vi "SO55 Ion Source Main.vi"() -> ()   [LabVIEW 2013]
panel:
  out "AnodeCurrentInd":dbl format="%#.3g"
  out "Anode Current":dbl(knob) scale=0.0..10.0
  out "GasInd":dbl format="%#.3g"
  out "Gasmeter":dbl(knob) scale=0.0..40.0
  in  "Gas":dbl(knob) min=0.0 max=40.0 step=0.1 scale=0.0..40.0
  in  "ExitBtn":bool
  in  "SetBtn":bool
  out "AnodeInd":dbl format="%#.3g"
  out "Anodemeter":dbl(knob) scale=0.0..250.0 scale format="%-#3.3p"
  in  "Anode":dbl(knob) min=0.0 max=250.0 step=1.0 scale=0.0..250.0
  out "OvenInd":dbl format="%#.3g"
  out "MagInd":dbl format="%#.3g"
  out "FilInd":dbl format="%#.3g"
  out "Ovenmeter":dbl(knob) scale=0.0..40.0
  out "Magmeter":dbl(knob) scale=0.0..40.0
  out "Filmeter":dbl(knob) scale=0.0..40.0 scale format="%-#3.3p"
  in  "Oven":dbl(knob) min=0.0 max=40.0 step=0.1 scale=0.0..40.0
  in  "Mag":dbl(knob) min=0.0 max=30.0 step=0.1 scale=0.0..40.0
  in  "Fil":dbl(knob) min=0.0 max=40.0 step=0.1 scale=0.0..40.0
  # "Magnet"
  # "Oven"
  # "Gas"
  # "Anode"
  # "Filament"
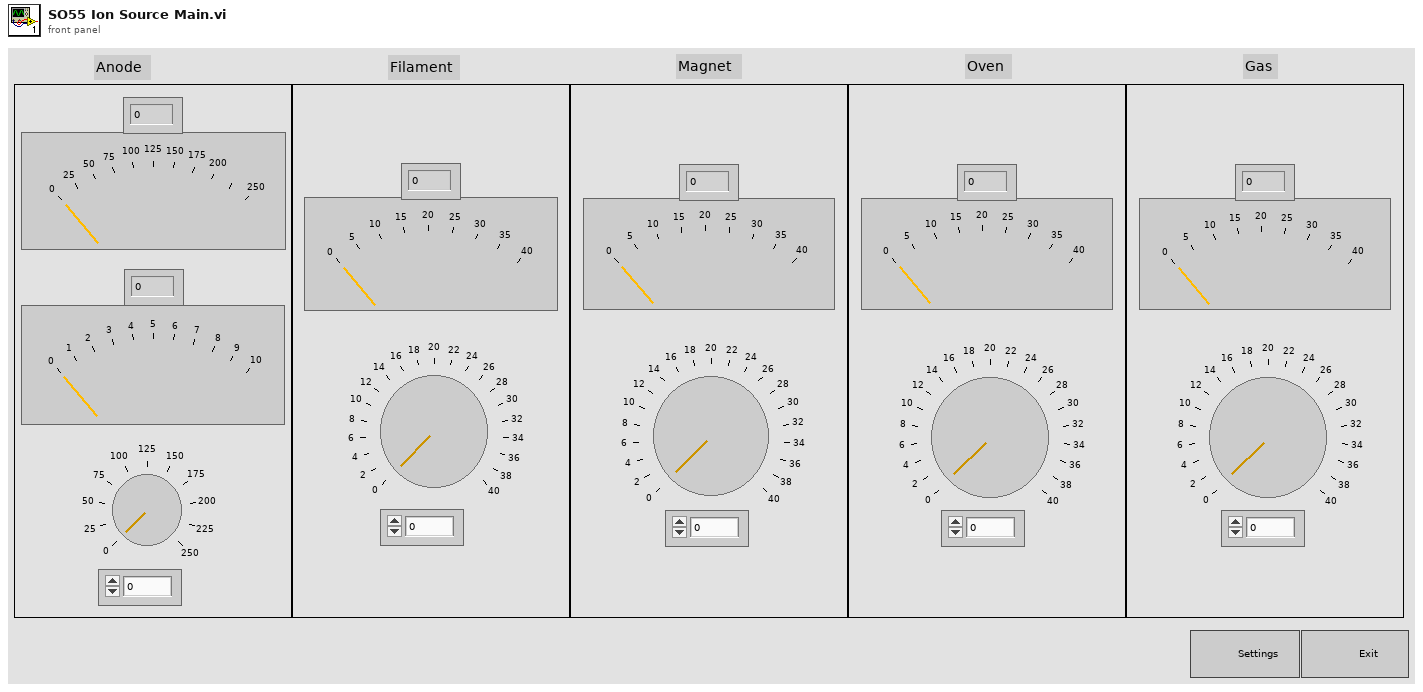
[diagram p1: front panel]
types:
  T1 = typedef "SO55 Settings Cluster.ctl" = cluster{"Input":cluster{"Anode Input Channel":tag, "Filament Input Channel":tag, "Magnet Input Channel":tag, "Oven Input Channel":tag, "Gas Input Channel":tag, "Input Rate":dbl, "Anode Current Input Channel":tag}, "Output":cluster{"Anode":cluster{"Anode Output Channel":tag, "Anode Step":dbl}, "Filament":cluster{"Filament Output Channel":tag, "Filament Step":dbl}, "Magnet":cluster{"Magnet Output Channel":tag, "Magnet Step":dbl}, "Oven":cluster{"Oven Output Channel":tag, "Oven Step":dbl}, "Gas":cluster{"Gas Output Channel":tag, "Gas Step":dbl}, "Output Rate":dbl}}
  T2 = enum8{"Enabled", "Disabled", "Disabled and Grayed Out"}
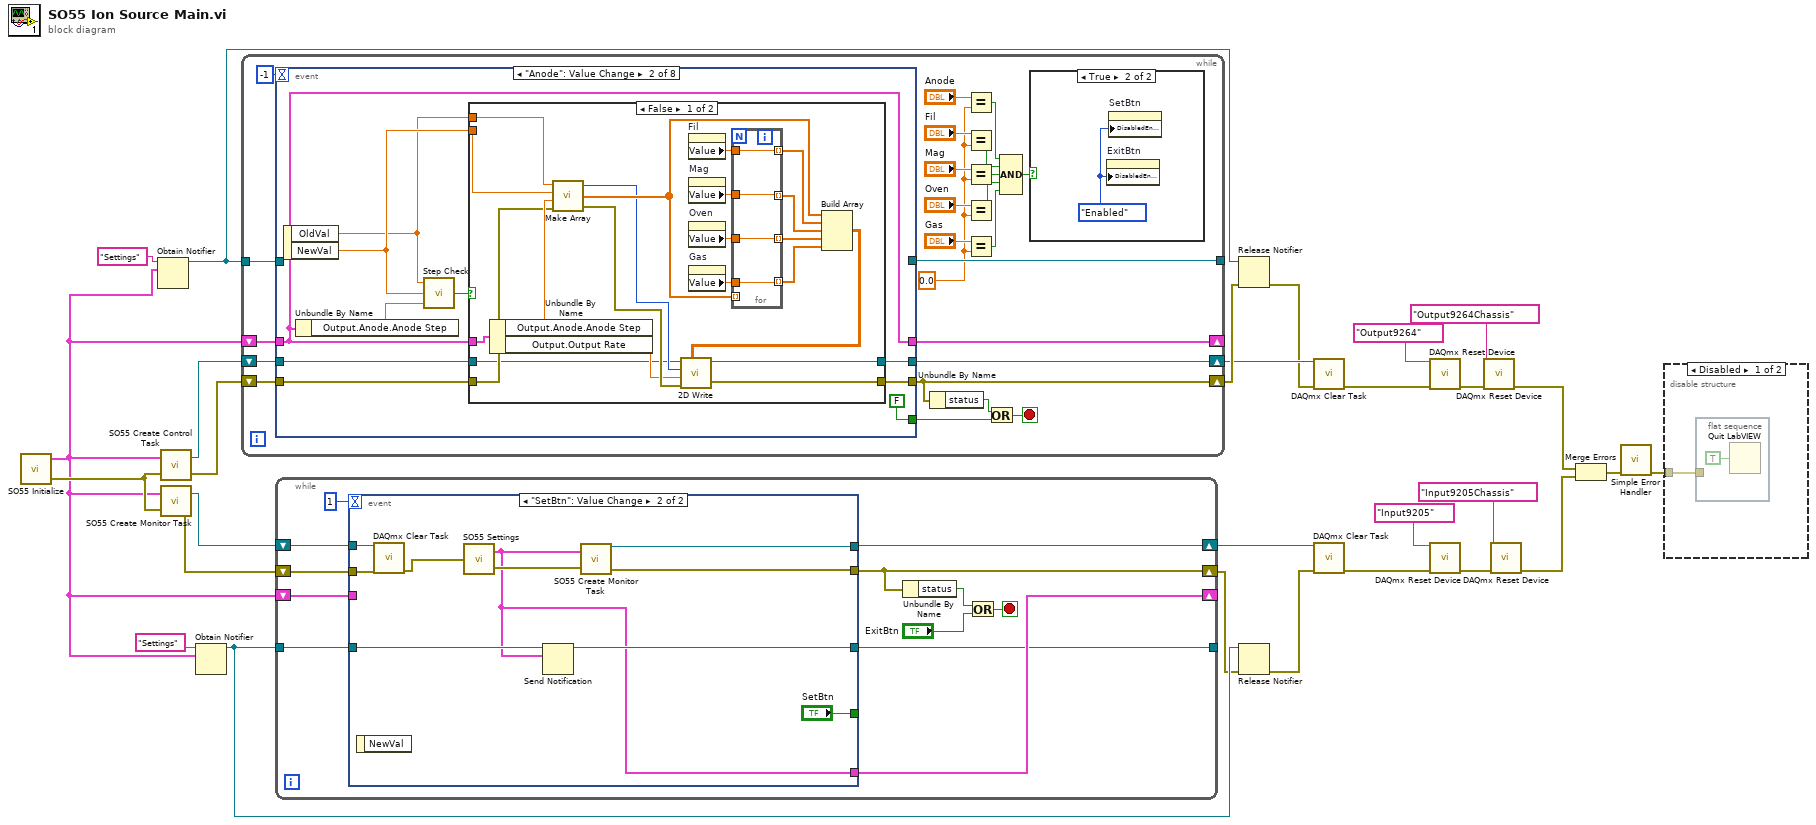
[diagram p0: block diagram]
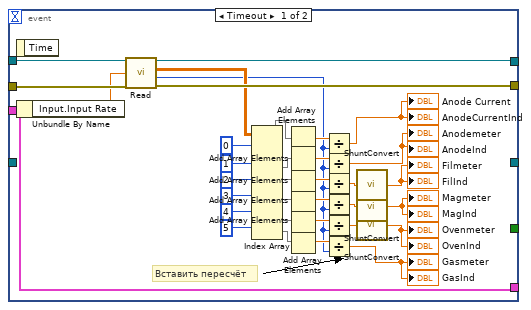
[diagram p3: hidden frame]
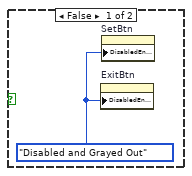
[diagram p4: hidden frame]
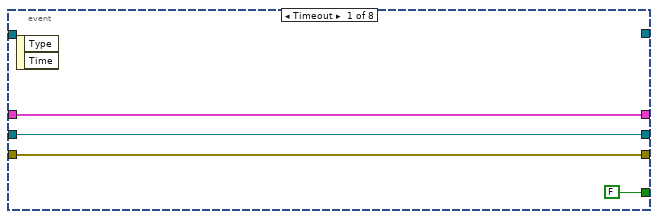
[diagram p5: hidden frame]
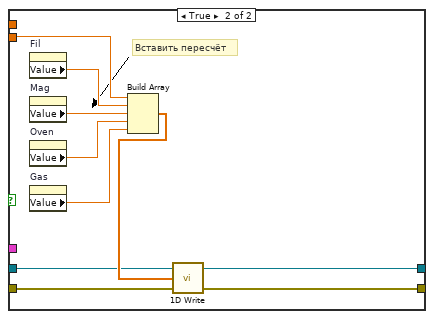
[diagram p6: hidden frame]
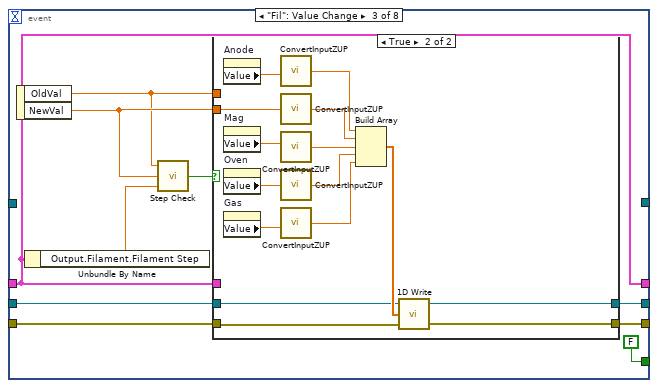
[diagram p7: hidden frame]
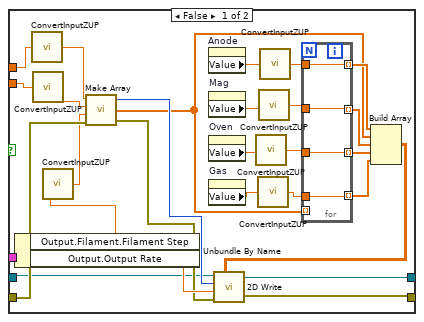
[diagram p8: hidden frame]
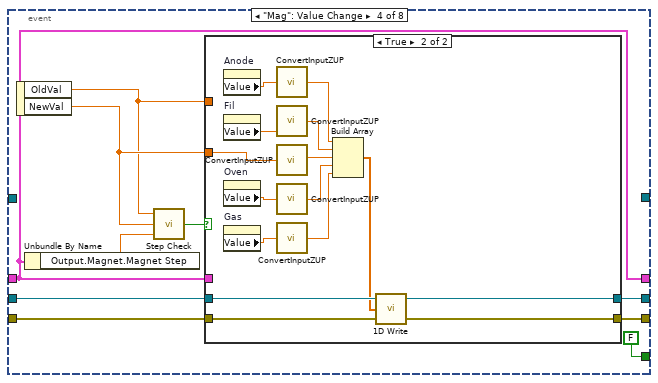
[diagram p9: hidden frame]
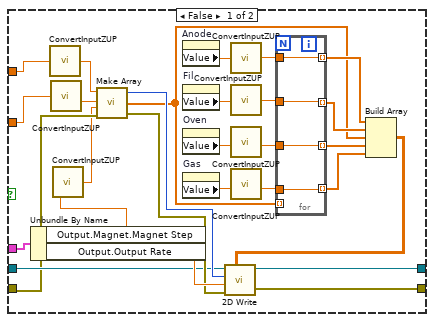
[diagram p10: hidden frame]
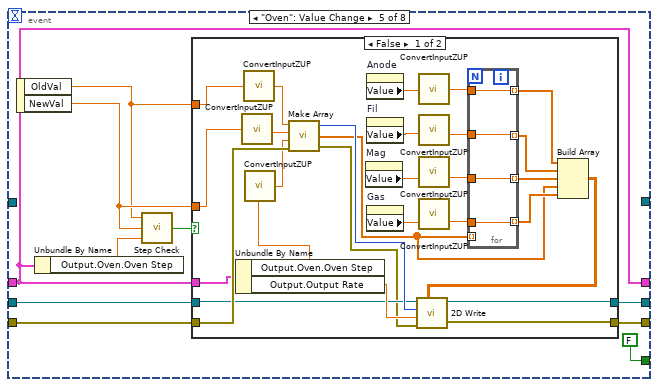
[diagram p11: hidden frame]
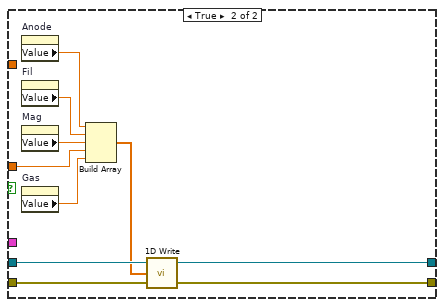
[diagram p12: hidden frame]
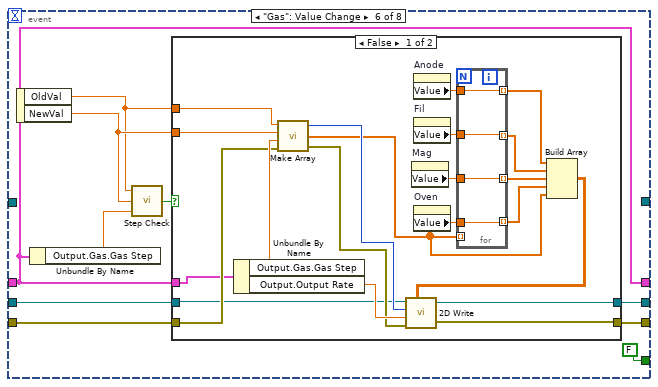
[diagram p13: hidden frame]
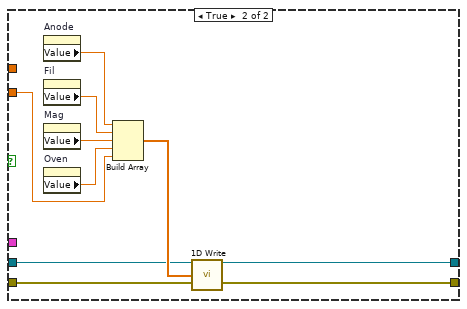
[diagram p14: hidden frame]
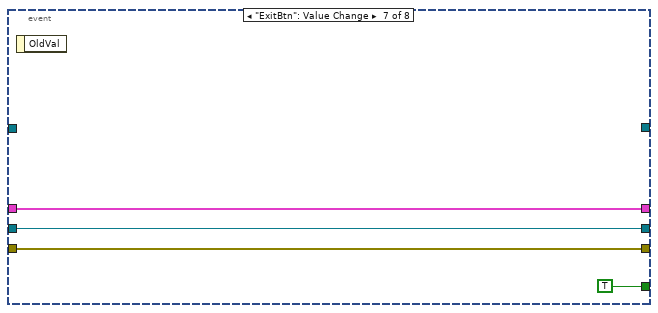
[diagram p15: hidden frame]
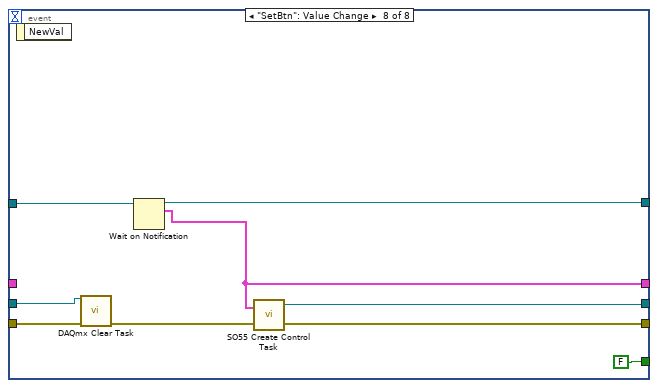
[diagram p16: hidden frame]
diagram:
  n1 = call "SO55 Initialize.vi"() -> ("error out"=w28:errorcluster, "Settings Out"=w1:T1)  [unwired: 1 in]
  n2 = Obtain Notifier(name (unnamed)="Settings", notification data type=w1) -> (notifier out=w3:refnum<notifier>)  [unwired: 2 in, 2 out]
  n3 = call "SO55 Create Control Task.vi"("error in"=w28, "Output"=w1) -> ("error out"=w24:errorcluster, "task out"=w25:refnum<k21>)
  n4 = call "SO55 Create Monitor Task.vi"("error in"=w28, "Input"=w1) -> ("error out"=w26:errorcluster, "task out"=w27:refnum<k21>)
  n5 = Obtain Notifier(name (unnamed)="Settings", notification data type=w1) -> (notifier out=w4:refnum<notifier>)  [unwired: 2 in, 2 out]
  n6 = while {
    shift-right: [w46] -> w21
    shift-left: w24 -> [w49]
    shift-right: [w51] -> w20
    shift-left: w25 -> [w50]
    shift-right: [w47] -> _
    shift-left: w1 -> [w48]
    tunnel: w3 -> [w42]
    tunnel: [w41] -> _
    stop <- w43 stop-if-true
    w35 = 0.0
    n7 = event shown="[1] \"Anode\": Value Change" {
      selector: _ -> [_ _ _ _ _ _ _ _]
      dyn-events: _ -> [_ _ _ _ _ _ _ _]
      timeout: -1 -> [_ _ _ _ _ _ _ _]
      tunnel: [w58 w66 w111 w165 w222 w274 w316 w321] -> w51
      tunnel: w50 -> [w58 w68 w113 w167 w224 w276 w316 w325]
      tunnel: [w57 w65 w110 w164 w221 w273 w315 w320] -> w46
      tunnel: w49 -> [w57 w67 w112 w166 w223 w275 w315 w326]
      tunnel: [w56 w59 w104 w161 w218 w270 w317 w319] -> w47
      tunnel: w48 -> [w56 w59 w104 w161 w218 w270 w317 _]
      tunnel: [FALSE FALSE FALSE FALSE FALSE FALSE TRUE FALSE] -> w44
      tunnel: w42 -> [_ _ _ _ _ _ _ w324]
      tunnel: [_ _ _ _ _ _ _ w323] -> w41
      event Timeout {
        n8 = event-data() -> ()  [unwired: 1 in, 2 out]
      }
      event "Anode": Value Change {
        n9 = event-data() -> ("OldVal"=w60:dbl, "NewVal"=w63:dbl)  [unwired: 1 in]
        n10 = Unbundle By Name(w59) -> ("Output.Anode.Anode Step"=w62:dbl)
        n11 = call "Step Check.vi"("Step"=w62, "New Value"=w63, "Old Value"=w60) -> ("Instant output"=w64:bool)
        n12 = case shown="False" w64 {
          tunnel: w63 -> [w87 w103]
          tunnel: w68 -> [w69 w97]
          tunnel: w67 -> [w85 w96]
          tunnel: [w71 w95] -> w66
          tunnel: [w70 w94] -> w65
          tunnel: w60 -> [w88 _]
          tunnel: w59 -> [w89 _]
          frame False {
            n13 = Unbundle By Name(w89) -> ("Output.Anode.Anode Step"=w86:dbl, "Output.Output Rate"=w72:dbl)
            n14 = call "Make Array.vi"("Error In"=w85, "Step"=w86, "New"=w87, "Old"=w88) -> ("Error Out"=w74:errorcluster, "Array"=w76:dbl[], "Samples"=w73:i32)
            n15 = property on="Fil" class="Knob (strict)"() -> ("Value"=w84:dbl)  [unwired: 2 in, 2 out]
            n16 = property on="Mag" class="Knob (strict)"() -> ("Value"=w83:dbl)  [unwired: 2 in, 2 out]
            n17 = property on="Oven" class="Knob (strict)"() -> ("Value"=w82:dbl)  [unwired: 2 in, 2 out]
            n18 = property on="Gas" class="Knob (strict)"() -> ("Value"=w81:dbl)  [unwired: 2 in, 2 out]
            n19 = for {
              tunnel: w84 -> [w93]
              tunnel: w83 -> [w92]
              tunnel: w76 -> [_] mode=indexing
              tunnel: w82 -> [w91]
              tunnel: w81 -> [w90]
              tunnel: [w93] -> w77 mode=indexing
              tunnel: [w92] -> w78 mode=indexing
              tunnel: [w91] -> w79 mode=indexing
              tunnel: [w90] -> w80 mode=indexing
            }
            n20 = Build Array(w76, w77, w78, w79, w80) -> (w75:dbl[][])
            n21 = call "2D Write.vi"("Task"=w69, "samples per channel"=w73, "rate"=w72, "Error In"=w74, "data"=w75) -> ("task out"=w71:refnum<k21>, "Error Out"=w70:errorcluster)
          }
          frame True {
            # "Вставить пересчёт"
            n22 = property on="Fil" class="Knob (strict)"() -> ("Value"=w99:dbl)  [unwired: 2 in, 2 out]
            n23 = property on="Mag" class="Knob (strict)"() -> ("Value"=w102:dbl)  [unwired: 2 in, 2 out]
            n24 = property on="Oven" class="Knob (strict)"() -> ("Value"=w101:dbl)  [unwired: 2 in, 2 out]
            n25 = property on="Gas" class="Knob (strict)"() -> ("Value"=w100:dbl)  [unwired: 2 in, 2 out]
            n26 = Build Array(w103, w99, w102, w101, w100) -> (w98:dbl[])
            n27 = call "1D Write.vi"("error in (no error)"=w96, "Data Array"=w98, "Task in"=w97) -> ("error out"=w94:errorcluster, "Task out"=w95:refnum<k21>)
          }
        }
      }
      event "Fil": Value Change {
        n28 = event-data() -> ("OldVal"=w105:dbl, "NewVal"=w107:dbl)  [unwired: 1 in]
        n29 = Unbundle By Name(w104) -> ("Output.Filament.Filament Step"=w108:dbl)
        n30 = call "Step Check.vi"("Step"=w108, "New Value"=w107, "Old Value"=w105) -> ("Instant output"=w109:bool)
        n31 = case shown="True" w109 {
          tunnel: w107 -> [w125 w153]
          tunnel: w113 -> [w130 w159]
          tunnel: w112 -> [w133 w158]
          tunnel: [w129 w157] -> w111
          tunnel: [w131 w156] -> w110
          tunnel: w104 -> [w128 _]
          tunnel: w105 -> [w127 _]
          frame False {
            n32 = Unbundle By Name(w128) -> ("Output.Filament.Filament Step"=w123:dbl, "Output.Output Rate"=w136:dbl)
            n33 = call "ConvertInputZUP.vi"("Current"=w127) -> ("ZUP input voltage"=w126:dbl)
            n34 = call "ConvertInputZUP.vi"("Current"=w125) -> ("ZUP input voltage"=w124:dbl)
            n35 = call "ConvertInputZUP.vi"("Current"=w123) -> ("ZUP input voltage"=w122:dbl)
            n36 = call "Make Array.vi"("Error In"=w133, "Step"=w122, "New"=w124, "Old"=w126) -> ("Error Out"=w132:errorcluster, "Array"=w134:dbl[], "Samples"=w137:i32)
            n37 = property on="Anode" class="Knob (strict)"() -> ("Value"=w114:dbl)  [unwired: 2 in, 2 out]
            n38 = property on="Mag" class="Knob (strict)"() -> ("Value"=w117:dbl)  [unwired: 2 in, 2 out]
            n39 = property on="Oven" class="Knob (strict)"() -> ("Value"=w119:dbl)  [unwired: 2 in, 2 out]
            n40 = property on="Gas" class="Knob (strict)"() -> ("Value"=w121:dbl)  [unwired: 2 in, 2 out]
            n41 = call "ConvertInputZUP.vi"("Current"=w119) -> ("ZUP input voltage"=w118:dbl)
            n42 = call "ConvertInputZUP.vi"("Current"=w121) -> ("ZUP input voltage"=w120:dbl)
            n43 = call "ConvertInputZUP.vi"("Current"=w117) -> ("ZUP input voltage"=w116:dbl)
            n44 = call "ConvertInputZUP.vi"("Current"=w114) -> ("ZUP input voltage"=w115:dbl)
            n45 = for {
              tunnel: w115 -> [w145]
              tunnel: w116 -> [w144]
              tunnel: w134 -> [_] mode=indexing
              tunnel: w118 -> [w143]
              tunnel: w120 -> [w142]
              tunnel: [w145] -> w135 mode=indexing
              tunnel: [w144] -> w139 mode=indexing
              tunnel: [w143] -> w140 mode=indexing
              tunnel: [w142] -> w141 mode=indexing
            }
            n46 = Build Array(w135, w134, w139, w140, w141) -> (w138:dbl[][])
            n47 = call "2D Write.vi"("Task"=w130, "samples per channel"=w137, "rate"=w136, "Error In"=w132, "data"=w138) -> ("task out"=w129:refnum<k21>, "Error Out"=w131:errorcluster)
          }
          frame True {
            n48 = property on="Anode" class="Knob (strict)"() -> ("Value"=w155:dbl)  [unwired: 2 in, 2 out]
            n49 = property on="Mag" class="Knob (strict)"() -> ("Value"=w151:dbl)  [unwired: 2 in, 2 out]
            n50 = property on="Oven" class="Knob (strict)"() -> ("Value"=w149:dbl)  [unwired: 2 in, 2 out]
            n51 = property on="Gas" class="Knob (strict)"() -> ("Value"=w147:dbl)  [unwired: 2 in, 2 out]
            n52 = call "ConvertInputZUP.vi"("Current"=w155) -> ("ZUP input voltage"=w154:dbl)
            n53 = call "ConvertInputZUP.vi"("Current"=w153) -> ("ZUP input voltage"=w152:dbl)
            n54 = call "ConvertInputZUP.vi"("Current"=w151) -> ("ZUP input voltage"=w150:dbl)
            n55 = call "ConvertInputZUP.vi"("Current"=w149) -> ("ZUP input voltage"=w148:dbl)
            n56 = call "ConvertInputZUP.vi"("Current"=w147) -> ("ZUP input voltage"=w146:dbl)
            n57 = Build Array(w154, w152, w150, w148, w146) -> (w160:dbl[])
            n58 = call "1D Write.vi"("error in (no error)"=w158, "Data Array"=w160, "Task in"=w159) -> ("error out"=w156:errorcluster, "Task out"=w157:refnum<k21>)
          }
        }
      }
      event "Mag": Value Change {
        n59 = event-data() -> ("OldVal"=w162:dbl, "NewVal"=w168:dbl)  [unwired: 1 in]
        n60 = Unbundle By Name(w161) -> ("Output.Magnet.Magnet Step"=w169:dbl)
        n61 = call "Step Check.vi"("Step"=w169, "New Value"=w168, "Old Value"=w162) -> ("Instant output"=w170:bool)
        n62 = case shown="True" w170 {
          tunnel: w168 -> [w181 w207]
          tunnel: w167 -> [w189 w217]
          tunnel: w166 -> [w188 w216]
          tunnel: [w191 w215] -> w165
          tunnel: [w190 w214] -> w164
          tunnel: w162 -> [w184 _]
          tunnel: w161 -> [w185 _]
          frame False {
            n63 = Unbundle By Name(w185) -> ("Output.Magnet.Magnet Step"=w180:dbl, "Output.Output Rate"=w194:dbl)
            n64 = call "ConvertInputZUP.vi"("Current"=w184) -> ("ZUP input voltage"=w183:dbl)
            n65 = call "ConvertInputZUP.vi"("Current"=w181) -> ("ZUP input voltage"=w182:dbl)
            n66 = call "ConvertInputZUP.vi"("Current"=w180) -> ("ZUP input voltage"=w179:dbl)
            n67 = call "Make Array.vi"("Error In"=w188, "Step"=w179, "New"=w182, "Old"=w183) -> ("Error Out"=w192:errorcluster, "Array"=w186:dbl[], "Samples"=w195:i32)
            n68 = property on="Anode" class="Knob (strict)"() -> ("Value"=w177:dbl)  [unwired: 2 in, 2 out]
            n69 = property on="Fil" class="Knob (strict)"() -> ("Value"=w176:dbl)  [unwired: 2 in, 2 out]
            n70 = property on="Oven" class="Knob (strict)"() -> ("Value"=w174:dbl)  [unwired: 2 in, 2 out]
            n71 = property on="Gas" class="Knob (strict)"() -> ("Value"=w172:dbl)  [unwired: 2 in, 2 out]
            n72 = call "ConvertInputZUP.vi"("Current"=w177) -> ("ZUP input voltage"=w178:dbl)
            n73 = call "ConvertInputZUP.vi"("Current"=w176) -> ("ZUP input voltage"=w175:dbl)
            n74 = call "ConvertInputZUP.vi"("Current"=w174) -> ("ZUP input voltage"=w173:dbl)
            n75 = call "ConvertInputZUP.vi"("Current"=w172) -> ("ZUP input voltage"=w171:dbl)
            n76 = for {
              tunnel: w178 -> [w202]
              tunnel: w175 -> [w201]
              tunnel: w186 -> [_] mode=indexing
              tunnel: w173 -> [w200]
              tunnel: w171 -> [w199]
              tunnel: [w202] -> w193 mode=indexing
              tunnel: [w201] -> w187 mode=indexing
              tunnel: [w200] -> w197 mode=indexing
              tunnel: [w199] -> w198 mode=indexing
            }
            n77 = Build Array(w193, w187, w186, w197, w198) -> (w196:dbl[][])
            n78 = call "2D Write.vi"("Task"=w189, "samples per channel"=w195, "rate"=w194, "Error In"=w192, "data"=w196) -> ("task out"=w191:refnum<k21>, "Error Out"=w190:errorcluster)
          }
          frame True {
            n79 = property on="Anode" class="Knob (strict)"() -> ("Value"=w212:dbl)  [unwired: 2 in, 2 out]
            n80 = property on="Fil" class="Knob (strict)"() -> ("Value"=w210:dbl)  [unwired: 2 in, 2 out]
            n81 = property on="Oven" class="Knob (strict)"() -> ("Value"=w206:dbl)  [unwired: 2 in, 2 out]
            n82 = property on="Gas" class="Knob (strict)"() -> ("Value"=w204:dbl)  [unwired: 2 in, 2 out]
            n83 = call "ConvertInputZUP.vi"("Current"=w212) -> ("ZUP input voltage"=w211:dbl)
            n84 = call "ConvertInputZUP.vi"("Current"=w210) -> ("ZUP input voltage"=w209:dbl)
            n85 = call "ConvertInputZUP.vi"("Current"=w207) -> ("ZUP input voltage"=w208:dbl)
            n86 = call "ConvertInputZUP.vi"("Current"=w206) -> ("ZUP input voltage"=w205:dbl)
            n87 = call "ConvertInputZUP.vi"("Current"=w204) -> ("ZUP input voltage"=w203:dbl)
            n88 = Build Array(w211, w209, w208, w205, w203) -> (w213:dbl[])
            n89 = call "1D Write.vi"("error in (no error)"=w216, "Data Array"=w213, "Task in"=w217) -> ("error out"=w214:errorcluster, "Task out"=w215:refnum<k21>)
          }
        }
      }
      event "Oven": Value Change {
        n90 = event-data() -> ("OldVal"=w219:dbl, "NewVal"=w225:dbl)  [unwired: 1 in]
        n91 = Unbundle By Name(w218) -> ("Output.Oven.Oven Step"=w226:dbl)
        n92 = call "Step Check.vi"("Step"=w226, "New Value"=w225, "Old Value"=w219) -> ("Instant output"=w227:bool)
        n93 = case shown="False" w227 {
          tunnel: w225 -> [w238 w268]
          tunnel: w224 -> [w246 w264]
          tunnel: w223 -> [w247 w263]
          tunnel: [w249 w262] -> w222
          tunnel: [w248 w261] -> w221
          tunnel: w219 -> [w240 _]
          tunnel: w218 -> [w245 _]
          frame False {
            n94 = Unbundle By Name(w245) -> ("Output.Oven.Oven Step"=w236:dbl, "Output.Output Rate"=w252:dbl)
            n95 = call "ConvertInputZUP.vi"("Current"=w238) -> ("ZUP input voltage"=w239:dbl)
            n96 = call "ConvertInputZUP.vi"("Current"=w240) -> ("ZUP input voltage"=w241:dbl)
            n97 = call "ConvertInputZUP.vi"("Current"=w236) -> ("ZUP input voltage"=w237:dbl)
            n98 = call "Make Array.vi"("Error In"=w247, "Step"=w237, "New"=w239, "Old"=w241) -> ("Error Out"=w244:errorcluster, "Array"=w242:dbl[], "Samples"=w253:i32)
            n99 = property on="Mag" class="Knob (strict)"() -> ("Value"=w231:dbl)  [unwired: 2 in, 2 out]
            n100 = property on="Anode" class="Knob (strict)"() -> ("Value"=w234:dbl)  [unwired: 2 in, 2 out]
            n101 = property on="Fil" class="Knob (strict)"() -> ("Value"=w233:dbl)  [unwired: 2 in, 2 out]
            n102 = property on="Gas" class="Knob (strict)"() -> ("Value"=w230:dbl)  [unwired: 2 in, 2 out]
            n103 = call "ConvertInputZUP.vi"("Current"=w234) -> ("ZUP input voltage"=w235:dbl)
            n104 = call "ConvertInputZUP.vi"("Current"=w233) -> ("ZUP input voltage"=w232:dbl)
            n105 = call "ConvertInputZUP.vi"("Current"=w231) -> ("ZUP input voltage"=w228:dbl)
            n106 = call "ConvertInputZUP.vi"("Current"=w230) -> ("ZUP input voltage"=w229:dbl)
            n107 = for {
              tunnel: w235 -> [w259]
              tunnel: w232 -> [w258]
              tunnel: w242 -> [_] mode=indexing
              tunnel: w228 -> [w257]
              tunnel: w229 -> [w256]
              tunnel: [w259] -> w251 mode=indexing
              tunnel: [w258] -> w250 mode=indexing
              tunnel: [w257] -> w243 mode=indexing
              tunnel: [w256] -> w255 mode=indexing
            }
            n108 = Build Array(w251, w250, w243, w242, w255) -> (w254:dbl[][])
            n109 = call "2D Write.vi"("Task"=w246, "samples per channel"=w253, "rate"=w252, "Error In"=w244, "data"=w254) -> ("task out"=w249:refnum<k21>, "Error Out"=w248:errorcluster)
          }
          frame True {
            n110 = property on="Anode" class="Knob (strict)"() -> ("Value"=w265:dbl)  [unwired: 2 in, 2 out]
            n111 = property on="Fil" class="Knob (strict)"() -> ("Value"=w266:dbl)  [unwired: 2 in, 2 out]
            n112 = property on="Mag" class="Knob (strict)"() -> ("Value"=w267:dbl)  [unwired: 2 in, 2 out]
            n113 = property on="Gas" class="Knob (strict)"() -> ("Value"=w269:dbl)  [unwired: 2 in, 2 out]
            n114 = Build Array(w265, w266, w267, w268, w269) -> (w260:dbl[])
            n115 = call "1D Write.vi"("error in (no error)"=w263, "Data Array"=w260, "Task in"=w264) -> ("error out"=w261:errorcluster, "Task out"=w262:refnum<k21>)
          }
        }
      }
      event "Gas": Value Change {
        n116 = event-data() -> ("OldVal"=w271:dbl, "NewVal"=w277:dbl)  [unwired: 1 in]
        n117 = Unbundle By Name(w270) -> ("Output.Gas.Gas Step"=w278:dbl)
        n118 = call "Step Check.vi"("Step"=w278, "New Value"=w277, "Old Value"=w271) -> ("Instant output"=w279:bool)
        n119 = case shown="False" w279 {
          tunnel: w277 -> [w285 w310]
          tunnel: w276 -> [w288 w308]
          tunnel: w275 -> [w289 w307]
          tunnel: [w291 w306] -> w274
          tunnel: [w290 w305] -> w273
          tunnel: w270 -> [w287 _]
          tunnel: w271 -> [w286 _]
          frame False {
            n120 = Unbundle By Name(w287) -> ("Output.Gas.Gas Step"=w300:dbl, "Output.Output Rate"=w297:dbl)
            n121 = call "Make Array.vi"("Error In"=w289, "Step"=w300, "New"=w285, "Old"=w286) -> ("Error Out"=w294:errorcluster, "Array"=w280:dbl[], "Samples"=w298:i32)
            n122 = property on="Mag" class="Knob (strict)"() -> ("Value"=w283:dbl)  [unwired: 2 in, 2 out]
            n123 = property on="Anode" class="Knob (strict)"() -> ("Value"=w296:dbl)  [unwired: 2 in, 2 out]
            n124 = property on="Fil" class="Knob (strict)"() -> ("Value"=w293:dbl)  [unwired: 2 in, 2 out]
            n125 = property on="Oven" class="Knob (strict)"() -> ("Value"=w284:dbl)  [unwired: 2 in, 2 out]
            n126 = for {
              tunnel: w296 -> [w304]
              tunnel: w293 -> [w303]
              tunnel: w280 -> [_] mode=indexing
              tunnel: w283 -> [w302]
              tunnel: w284 -> [w301]
              tunnel: [w304] -> w295 mode=indexing
              tunnel: [w303] -> w292 mode=indexing
              tunnel: [w302] -> w282 mode=indexing
              tunnel: [w301] -> w281 mode=indexing
            }
            n127 = Build Array(w295, w292, w282, w281, w280) -> (w299:dbl[][])
            n128 = call "2D Write.vi"("Task"=w288, "samples per channel"=w298, "rate"=w297, "Error In"=w294, "data"=w299) -> ("task out"=w291:refnum<k21>, "Error Out"=w290:errorcluster)
          }
          frame True {
            n129 = property on="Anode" class="Knob (strict)"() -> ("Value"=w313:dbl)  [unwired: 2 in, 2 out]
            n130 = property on="Fil" class="Knob (strict)"() -> ("Value"=w314:dbl)  [unwired: 2 in, 2 out]
            n131 = property on="Mag" class="Knob (strict)"() -> ("Value"=w312:dbl)  [unwired: 2 in, 2 out]
            n132 = property on="Oven" class="Knob (strict)"() -> ("Value"=w311:dbl)  [unwired: 2 in, 2 out]
            n133 = Build Array(w313, w314, w312, w311, w310) -> (w309:dbl[])
            n134 = call "1D Write.vi"("error in (no error)"=w307, "Data Array"=w309, "Task in"=w308) -> ("error out"=w305:errorcluster, "Task out"=w306:refnum<k21>)
          }
        }
      }
      event "ExitBtn": Value Change {
        n135 = event-data() -> ()  [unwired: 1 in, 1 out]
      }
      event "SetBtn": Value Change {
        n136 = event-data() -> ()  [unwired: 1 in, 1 out]
        n137 = call <vilib>:"DAQmx Clear Task.vi"("task in"=w325, "error in"=w326) -> ("error out"=w322:errorcluster)  [unwired: 13 in]
        n138 = Wait on Notification(notifier=w324) -> (notifier out=w323:refnum<notifier>, notification=w319:T1)  [unwired: 3 in, 2 out]
        n139 = call "SO55 Create Control Task.vi"("error in"=w322, "Output"=w319) -> ("error out"=w320:errorcluster, "task out"=w321:refnum<k21>)
      }
    }
    n140 = Unbundle By Name(w46) -> ("status"=w45:bool)
    n141 = Equal?(x="Anode", y=w35) -> (x = y?=w34:bool)
    n142 = Equal?(x="Fil", y=w35) -> (x = y?=w33:bool)
    n143 = Equal?(x="Mag", y=w35) -> (x = y?=w32:bool)
    n144 = Equal?(x="Oven", y=w35) -> (x = y?=w31:bool)
    n145 = Equal?(x="Gas", y=w35) -> (x = y?=w30:bool)
    n146 = Or(x=w45, y=w44) -> (x .or. y?=w43:bool)
    n147 = Compound Arithmetic op=AND(w34, w33, w32, w31, w30) -> (w29:bool)
    n148 = case shown="True" w29 {
      frame False {
        w53 = T2."Disabled and Grayed Out" ("Disabled")
        n149 = property on="ExitBtn" class="Bool"("DisabledEnum"=w53) -> ()  [unwired: 2 in, 2 out]
        n150 = property on="SetBtn" class="Bool"("DisabledEnum"=w53) -> ()  [unwired: 2 in, 2 out]
      }
      frame True {
        w54 = T2."Enabled" ("Disabled")
        n151 = property on="ExitBtn" class="Bool"("DisabledEnum"=w54) -> ()  [unwired: 2 in, 2 out]
        n152 = property on="SetBtn" class="Bool"("DisabledEnum"=w54) -> ()  [unwired: 2 in, 2 out]
      }
    }
  }
  n153 = while {
    shift-right: [w333] -> w2
    shift-left: w26 -> [w337]
    shift-right: [w335] -> w18
    shift-left: w27 -> [w338]
    shift-right: [w334] -> _
    shift-left: w1 -> [w336]
    tunnel: w4 -> [w329]
    tunnel: [w328] -> _
    stop <- w330 stop-if-true
    n154 = event shown="[1] \"SetBtn\": Value Change" {
      selector: _ -> [_ _]
      dyn-events: _ -> [_ _]
      timeout: 1 -> [_ _]
      tunnel: [_ "SetBtn"] -> _
      tunnel: w338 -> [w374 w383]
      tunnel: w337 -> [w373 w382]
      tunnel: w336 -> [w352 _]
      tunnel: [w371 w377] -> w335
      tunnel: [w370 w376] -> w333
      tunnel: [w352 w375] -> w334
      tunnel: w329 -> [_ w380]
      tunnel: [_ w379] -> w328
      event Timeout {
        # "Вставить пересчёт"
        n155 = event-data() -> ()  [unwired: 1 in, 1 out]
        n156 = Unbundle By Name(w352) -> ("Input.Input Rate"=w372:dbl)
        n157 = call "Read.vi"("Task in"=w374, "Input Rate"=w372, "error in (no error)"=w373) -> ("Task out"=w371:refnum<k21>, "data"=w357:dbl[][], "samples"=w348:i32, "error out"=w370:errorcluster)
        n158 = Index Array(array=w357, index (row) #1=0 ("index (row)"), index (row) #2=1 ("index (row)"), index (row) #3=2 ("index (row)"), index (row) #4=3 ("index (row)"), index (row) #5=4 ("index (row)"), index (row) #6=5 ("index (row)")) -> (element #1=w350:dbl[], element #2=w365:dbl[], element #3=w364:dbl[], element #4=w363:dbl[], element #5=w362:dbl[], element #6=w355:dbl[])  [unwired: 6 in]
        n159 = Add Array Elements(numeric array=w350) -> (sum=w349:dbl)
        n160 = Add Array Elements(numeric array=w365) -> (sum=w361:dbl)
        n161 = Add Array Elements(numeric array=w364) -> (sum=w360:dbl)
        n162 = Add Array Elements(numeric array=w363) -> (sum=w359:dbl)
        n163 = Add Array Elements(numeric array=w362) -> (sum=w358:dbl)
        n164 = Add Array Elements(numeric array=w355) -> (sum=w354:dbl)
        n165 = Divide(x=w349, y=w348) -> (x/y=→"Anode Current" →"AnodeCurrentInd":dbl)
        n166 = Divide(x=w361, y=w348) -> (x/y=→"Anodemeter" →"AnodeInd":dbl)
        n167 = Divide(x=w360, y=w348) -> (x/y=w345:dbl)
        n168 = Divide(x=w359, y=w348) -> (x/y=w343:dbl)
        n169 = Divide(x=w358, y=w348) -> (x/y=w341:dbl)
        n170 = Divide(x=w354, y=w348) -> (x/y=→"Gasmeter" →"GasInd":dbl)
        n171 = call "ShuntConvert.vi"("Potential drop"=w345) -> ("Current"=→"Filmeter" →"FilInd":dbl)
        n172 = call "ShuntConvert.vi"("Potential drop"=w343) -> ("Current"=→"Magmeter" →"MagInd":dbl)
        n173 = call "ShuntConvert.vi"("Potential drop"=w341) -> ("Current"=→"Ovenmeter" →"OvenInd":dbl)
      }
      event "SetBtn": Value Change {
        n174 = event-data() -> ()  [unwired: 1 in, 1 out]
        n175 = call <vilib>:"DAQmx Clear Task.vi"("task in"=w383, "error in"=w382) -> ("error out"=w381:errorcluster)  [unwired: 13 in]
        n176 = call "SO55 Settings.vi"("Error In"=w381) -> ("Settings Out"=w375:T1, "Error Out"=w378:errorcluster)
        n177 = Send Notification(notification=w375, notifier=w380) -> (notifier out=w379:refnum<notifier>)  [unwired: 1 in, 1 out]
        n178 = call "SO55 Create Monitor Task.vi"("error in"=w378, "Input"=w375) -> ("error out"=w376:errorcluster, "task out"=w377:refnum<k21>)
      }
    }
    n179 = Unbundle By Name(w333) -> ("status"=w332:bool)
    n180 = Or(x=w332, y="ExitBtn") -> (x .or. y?=w330:bool)
  }
  n181 = Release Notifier(notifier=w3, error in (no error)=w21) -> (error out=w19:errorcluster)  [unwired: 1 in, 2 out]
  n182 = Release Notifier(notifier=w4, error in (no error)=w2) -> (error out=w17:errorcluster)  [unwired: 1 in, 2 out]
  n183 = call <vilib>:"DAQmx Clear Task.vi"("task in"=w20, "error in"=w19) -> ("error out"=w16:errorcluster)  [unwired: 13 in]
  n184 = call <vilib>:"DAQmx Clear Task.vi"("task in"=w18, "error in"=w17) -> ("error out"=w13:errorcluster)  [unwired: 13 in]
  n185 = call <vilib>:"DAQmx Reset Device.vi"("device in"=tag "Output9264", "error in"=w16) -> ("error out"=w10:errorcluster)  [unwired: 13 in]
  n186 = call <vilib>:"DAQmx Reset Device.vi"("device in"=tag "Input9205", "error in"=w13) -> ("error out"=w7:errorcluster)  [unwired: 13 in]
  n187 = call <vilib>:"DAQmx Reset Device.vi"("device in"=tag "Output9264Chassis", "error in"=w10) -> ("error out"=w9:errorcluster)  [unwired: 13 in]
  n188 = call <vilib>:"DAQmx Reset Device.vi"("device in"=tag "Input9205Chassis", "error in"=w7) -> ("error out"=w6:errorcluster)  [unwired: 13 in]
  n189 = Merge Errors(w9, w6) -> (w12:errorcluster)
  n190 = call <vilib>:"Simple Error Handler.vi"("error in (no error)"=w12) -> ("error out"=w11:errorcluster)  [unwired: 4 in, 4 out]
  n191 = disable-structure shown="Disabled" {
    disable-tunnel: w11 -> [w385 _]
    frame Disabled {
      n192 = flat-sequence {
        tunnel: w385 -> [_]
        frame #0 {
          n193 = Quit LabVIEW(quit? (T)=TRUE) -> ()
        }
      }
    }
    frame Enabled {
    }
  }
